vi "Configure RJDJ Mode.vi"(8 "error in (no error)":errorcluster, 9 "Unit Interval Count (0)":i32, 10 "Measurement Mode (0: Tie)":i32(ring) items=["Tie", "Period", "Unit Interval Number"], 11 "VISA resource name":refnum<visa-resource-name>) -> (0 "error out":errorcluster, 3 "VISA resource name out":refnum<visa-resource-name>)   [LabVIEW 2020, in "Agilent 90000 Series.lvlib"]
doc: "Configures the RJDJ measurement mode.\n\n<B>Note:</B>\nThis VI is only available when the N5400A/N5401A Software is installed."
uses:
  Agilent 90000 Series.lvlib
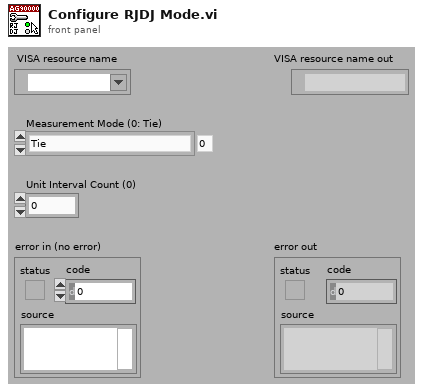
[diagram p1: front panel]
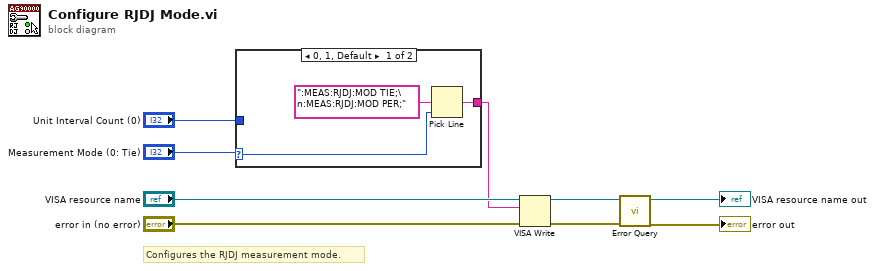
[diagram p0: block diagram]
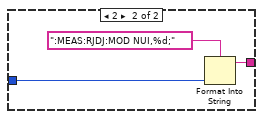
[diagram p2: hidden frame]
diagram:
  # "Configures the RJDJ measurement mode."
  n1 = case shown="0, 1, Default" "Measurement Mode (0: Tie)" {
    selector: "Measurement Mode (0: Tie)" -> [w11 _]
    tunnel: "Unit Interval Count (0)" -> [_ w14]
    tunnel: [w10 w13] -> w1
    frame 0, 1, Default {
      n2 = Pick Line(multi-line string=":MEAS:RJDJ:MOD TIE;\n:MEAS:RJDJ:MOD PER;", line index=w11) -> (output string=w10:string)  [unwired: 1 out]
    }
    frame 2 {
      n3 = Format Into String(format string=":MEAS:RJDJ:MOD NUI,%d;", w14) -> (resulting string=w13:string)  [unwired: 2 in, 1 out]
    }
  }
  n4 = VISA Write(VISA resource name="VISA resource name", write buffer=w1, error in (no error)="error in (no error)") -> (VISA resource name out=w7:refnum<visa-resource-name>, error out=w6:errorcluster)  [unwired: 1 out]
  n5 = call "Error Query.vi"("error in (no error)"=w6, "VISA resource name"=w7) -> ("error out"=→"error out":errorcluster, "VISA resource name out"=→"VISA resource name out":refnum<visa-resource-name>)  [unwired: 8 out]
